vi "Handle Error.vi"(0 "reference in":refnum<class "PM_Group.lvclass">, 11 "error in (no error)":errorcluster) -> (4 "reference out":refnum<class "PM_Group.lvclass">, 15 "error out":errorcluster)   [LabVIEW 2019, in "PM_Group.lvclass"]
uses:
  PM_Group.lvclass
  PM_Group.lvclass/PM_Group.ctl
  TypeDef/State PMG.ctl
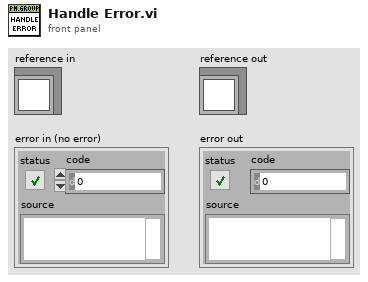
[diagram p1: front panel]
types:
  T1 = typedef "State PMG.ctl" = enum16{"NOT READY", "IDLE", "ACTIVE", "ERROR"}
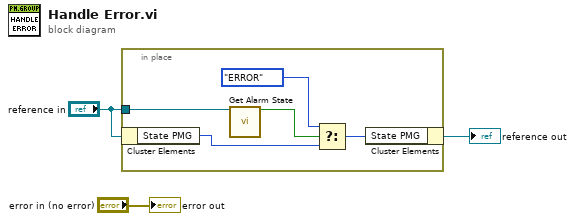
[diagram p0: block diagram]
diagram:
  n1 = in-place {
    in-place-border: "reference in" -> [w8]
    n2 = in-place-cluster #1("reference in") -> ("State PMG"=w6:T1)
    n3 = call "Get Alarm State.vi"("reference in"=w8) -> ("alarm state"=w7:bool)  [unwired: 14 in]
    n4 = Select(t=State_PMG."ERROR", s=w7, f=w6) -> (s? t:f=w5:T1)
    n5 = in-place-cluster #1("State PMG"=w5) -> (→"reference out":refnum<class "PM_Group.lvclass">)
  }
  "error out" <- "error in (no error)"
